vi "SetPiezoTriangularWave.vi"(5 "Período":sgl=20.0, 7 "lMode":i32=2, 8 "error in (no error)":errorcluster, 9 "amplitude":dbl=75.0, 10 "#Ciclos":i32=1, 11 "MG17Piezo in":refnum<k7>) -> (0 "error out":errorcluster, 3 "MG17Piezo out":refnum<k7>)   [LabVIEW 2014]
panel:
  in  "pfVoltage in":sgl
  # "#1-Ondas continuas(Desconsiderar # de ciclos)\n#2-Ciclos determinados"
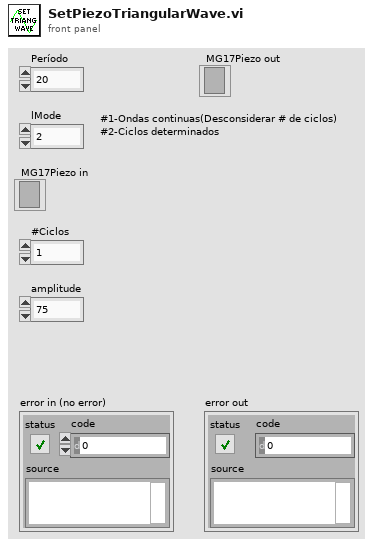
[diagram p1: front panel]
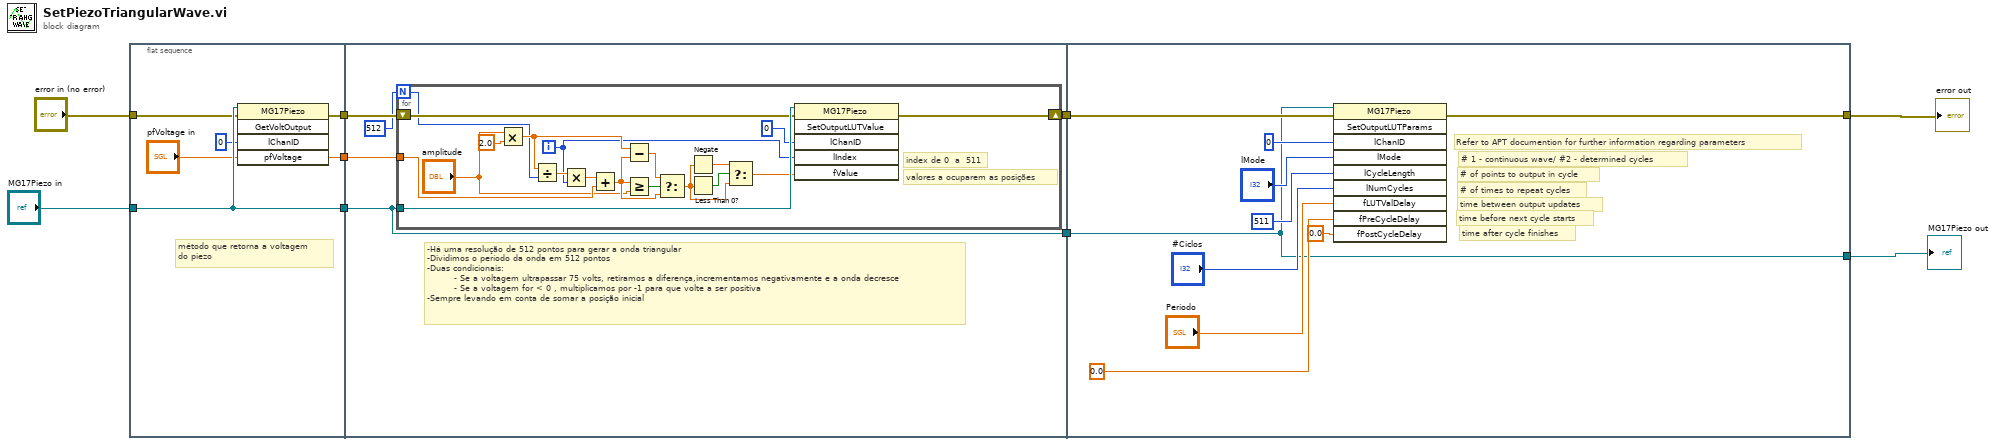
[diagram p0: block diagram]
diagram:
  # "Refer to APT documention for further information regarding parameters"
  n1 = flat-sequence {
    tunnel: "error in (no error)" -> [w14]
    tunnel: "MG17Piezo in" -> [w15]
    tunnel: [w15] -> w9
    tunnel: [w13] -> w8
    tunnel: [w10] -> w7
    tunnel: [w19] -> w6
    tunnel: [w20] -> w5
    tunnel: w9 -> [w19]
    tunnel: w8 -> [w18]
    tunnel: w7 -> [w17]
    tunnel: w6 -> [w41]
    tunnel: w5 -> [w48]
    tunnel: [w41] -> w3
    tunnel: [w40] -> w4
    frame #0 {
      # "método que retorna a voltagem \ndo piezo"
      n2 = invoke class="MG17Piezo" method="GetVoltOutput"(reference=w15, error in=w14, "lChanID"=0, "pfVoltage"="pfVoltage in") -> (error out=w13:errorcluster, "pfVoltage"=w10:sgl)  [unwired: 1 in, 3 out]
    }
    frame #1 {
      # "-Há uma resolução de 512 pontos para gerar a onda triangular\n-Dividimos o período da onda em 512 pontos \n-Duas condicionais:\n         - Se a voltagem ultrapassar 75 volts, retiramos a diferença,incrementamos negativamente e a onda decresce\n         - Se a voltagem for < 0 , multiplicamos por -1 para que volte a ser positiva\n-Sempre levando em conta de somar a posição inicial"
      n3 = for {
        N: 512 -> [w23]
        tunnel: w19 -> [w38]
        tunnel: w17 -> [w24]
        shift-right: [w39] -> w20
        shift-left: w18 -> [w37]
        i -> [w21]
        # "valores a ocuparem as posições"
        # "index de 0  a  511"
        n4 = Multiply(x="amplitude", y=2.0) -> (x*y=w26:dbl)
        n5 = Divide(x=w26, y=w23) -> (x/y=w35:dbl)
        n6 = Multiply(x=w35, y=w21) -> (x*y=w34:dbl)
        n7 = Add(x=w34, y=w24) -> (x+y=w31:dbl)
        n8 = Subtract(x=w26, y=w31) -> (x-y=w30:dbl)
        n9 = Greater Or Equal?(x=w31, y="amplitude") -> (x >= y?=w32:bool)
        n10 = Select(t=w30, s=w32, f=w31) -> (s? t:f=w28:dbl)
        n11 = Negate(x=w28) -> (-x=w27:dbl)
        n12 = Less Than 0?(x=w28) -> (x < 0?=w29:bool)
        n13 = Select(t=w27, s=w29, f=w28) -> (s? t:f=w25:dbl)
        n14 = invoke class="MG17Piezo" method="SetOutputLUTValue"(reference=w38, error in=w37, "lChanID"=0, "lIndex"=w21, "fValue"=w25) -> (error out=w39:errorcluster)  [unwired: 1 in, 5 out]
      }
    }
    frame #2 {
      # "time after cycle finishes"
      # "time before next cycle starts"
      # "time between output updates"
      # "# of times to repeat cycles"
      # "# of points to output in cycle"
      # "# 1 - continuous wave/ #2 - determined cycles"
      n15 = invoke class="MG17Piezo" method="SetOutputLUTParams"(reference=w41, error in=w48, "lChanID"=0, "lMode"="lMode", "lCycleLength"=511, "lNumCycles"="#Ciclos", "fLUTValDelay"="Período", "fPreCycleDelay"=sgl 0.0, "fPostCycleDelay"=sgl 0.0) -> (error out=w40:errorcluster)  [unwired: 1 in, 9 out]
    }
  }
  "error out" <- w4
  "MG17Piezo out" <- w3
